vi "AddNode.vi"(8 "error in (no error)":errorcluster, 9 "DirectedGraphMapNode.lvclass":refnum<class "NI_Robotics_DirectedGraphMapNode.lvclass">, 10 "Name":string, 11 "DirectedGraphWorldMap in":refnum<class "NI_Robotics_DirectedGraphWorldMap.lvclass">) -> (0 "error out":errorcluster, 2 "Already exists":bool, 3 "DirectedGraphWorldMap out":refnum<class "NI_Robotics_DirectedGraphWorldMap.lvclass">)   [LabVIEW 2017, in "NI_Robotics_DirectedGraphWorldMap.lvclass"]
uses:
  <vilib>/robotics/Navigation/shared/WorldMap/DirectedGraphWorldMap/NI_Robotics_DirectedGraphWorldMap.lvclass
  <vilib>/robotics/Navigation/shared/MapNode/DirectedGraphMapNode/NI_Robotics_DirectedGraphMapNode.lvclass
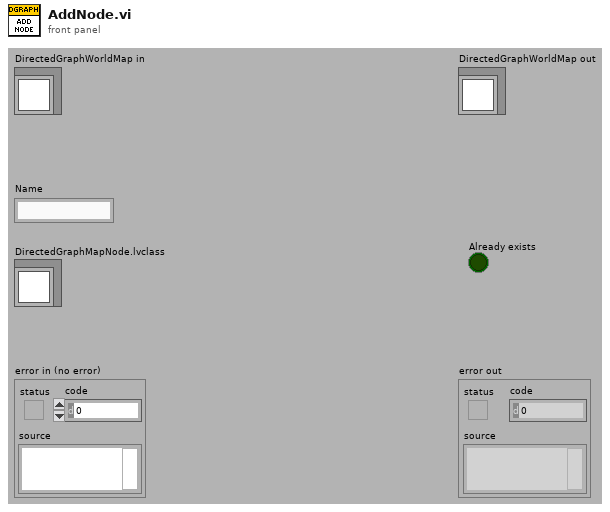
[diagram p1: front panel]
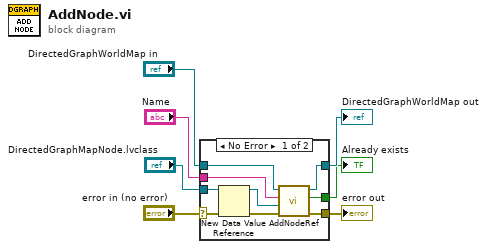
[diagram p0: block diagram]
diagram:
  n1 = case shown="No Error" "error in (no error)" {
    selector: "error in (no error)" -> [w16 w18]
    tunnel: [w14 w18] -> w6
    tunnel: [w11 w17] -> w4
    tunnel: "DirectedGraphWorldMap in" -> [w12 w17]
    tunnel: "DirectedGraphMapNode.lvclass" -> [w9 _]
    tunnel: "Name" -> [w10 _]
    tunnel: [w8 _] -> w1
    frame No Error {
      n2 = New Data Value Reference(data value=w9, error in=w16) -> (data value reference=w13:refnum<data-value>, error out=w15:errorcluster)
      n3 = call-dynamic "AddNodeRef.vi"("error in (no error)"=w15, "New node ref"=w13, "Node Name"=w10, "DirectedGraphWorldMap in"=w12) -> ("error out"=w14:errorcluster, "Already exists"=w8:bool, "DirectedGraphWorldMap out"=w11:refnum<class "NI_Robotics_DirectedGraphWorldMap.lvclass">)  [unwired: 5 in]
    }
    frame Error {
    }
  }
  "error out" <- w6
  "DirectedGraphWorldMap out" <- w4
  "Already exists" <- w1
